vi "Add Nonempty String Property.vi"(7 "Property":string, 10 "Value":string, 11 "String in":string) -> (3 "String":string)   [LabVIEW 2020, in "JWT.lvlib" / "JWT.lvclass"]
uses:
  JWT.lvclass
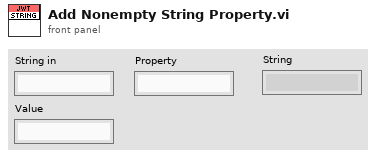
[diagram p1: front panel]
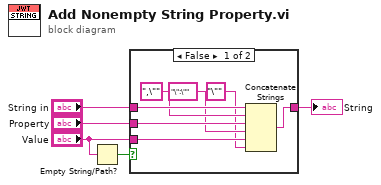
[diagram p0: block diagram]
diagram:
  n1 = Empty String/Path?(string/path="Value") -> (empty?=w4:bool)
  n2 = case shown="False" w4 {
    tunnel: "String in" -> [w12 w13]
    tunnel: "Value" -> [w8 _]
    tunnel: "Property" -> [w10 _]
    tunnel: [w6 w13] -> w1
    frame False {
      n3 = Concatenate Strings(w12, ",\"" ("string"), w10, "\":\"" ("string"), w8, "\"" ("string")) -> (w6:string)
    }
    frame True {
    }
  }
  "String" <- w1
